vi "Write Menu Reference.vi"(8 "error in (no error)":errorcluster, 10 "Menu Reference":refnum<k9>, 11 "Front Panel Menu in":refnum<class "Front Panel Menu.lvclass">) -> (0 "error out":errorcluster, 3 "Front Panel Menu out":refnum<class "Front Panel Menu.lvclass">)   [LabVIEW 2024, in "Front Panel Menu.lvclass"]
uses:
  Front Panel Menu.lvclass
  Front Panel Menu.lvclass/Front Panel Menu.ctl
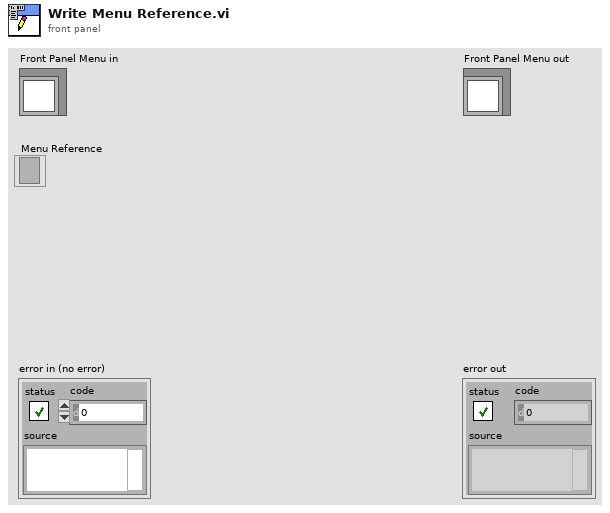
[diagram p1: front panel]
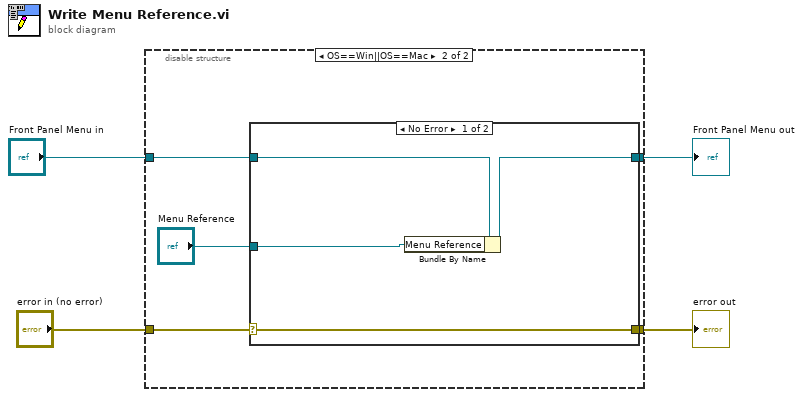
[diagram p0: block diagram]
diagram:
  n1 = disable-structure shown="OS==Win||OS==Mac" {
    disable-tunnel: "error in (no error)" -> [w5 w10]
    disable-tunnel: [w5 w9] -> w3
    disable-tunnel: "Front Panel Menu in" -> [w6 w11]
    disable-tunnel: [w6 w8] -> w1
    frame condition #0 {
    }
    frame condition #1 (active) {
      n2 = case shown="No Error" w10 {
        selector: w10 -> [w15 w16]
        tunnel: [w15 w16] -> w9
        tunnel: [w13 w17] -> w8
        tunnel: w11 -> [w14 w17]
        tunnel: "Menu Reference" -> [w12 _]
        frame No Error {
          n3 = Bundle By Name(cluster=w14, "Menu Reference"=w12) -> (w13:refnum<class "Front Panel Menu.lvclass">)
        }
        frame Error {
        }
      }
    }
  }
  "error out" <- w3
  "Front Panel Menu out" <- w1
